vi "Clear Tree.vi"(8 "error in":errorcluster, 11 "reference":refnum<vi>) -> (0 "error out":errorcluster, 3 "reference out":refnum<vi>)   [LabVIEW 2019, in "Report Viewer.lvlib" / "Report Viewer.lvclass"]
uses:
  Report Viewer.lvclass
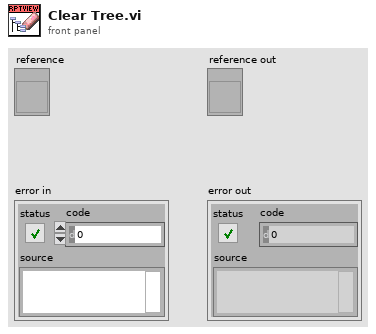
[diagram p1: front panel]
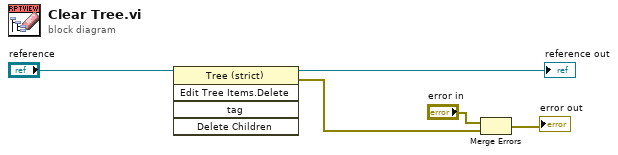
[diagram p0: block diagram]
diagram:
  n1 = invoke class="Tree (strict)" method="Edit Tree Items.Delete"(reference="reference") -> (reference out=→"reference out":refnum<vi>, error out=w5:errorcluster)  [unwired: 4 in, 3 out]
  n2 = Merge Errors("error in", w5) -> (→"error out":errorcluster)
